vi "Write Logger.vi"(8 "error in (no error)":errorcluster, 10 "Logger":refnum<class "Logger.lvclass">, 11 "LoggingActor in":refnum<class "LoggingActor.lvclass">) -> (0 "error out":errorcluster, 3 "LoggingActor out":refnum<class "LoggingActor.lvclass">)   [LabVIEW 2022 SP3, in "LoggingActor.lvlib" / "LoggingActor.lvclass"]
uses:
  LoggingActor.lvclass
  LoggingActor.lvclass/LoggingActor.ctl
  Logger/Source/Logger/Logger.lvclass
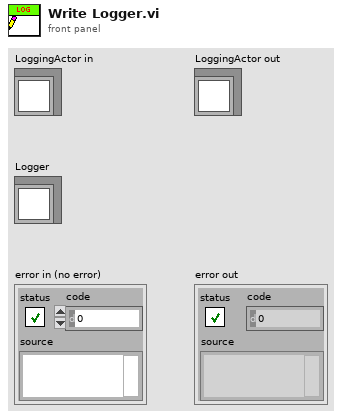
[diagram p1: front panel]
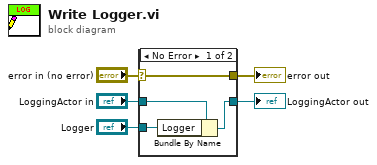
[diagram p0: block diagram]
diagram:
  n1 = case shown="No Error" "error in (no error)" {
    selector: "error in (no error)" -> [w9 w10]
    tunnel: [w9 w10] -> w4
    tunnel: [w7 w11] -> w2
    tunnel: "LoggingActor in" -> [w8 w11]
    tunnel: "Logger" -> [w6 _]
    frame No Error {
      n2 = Bundle By Name(cluster=w8, "Logger"=w6) -> (w7:refnum<class "LoggingActor.lvclass">)
    }
    frame Error {
    }
  }
  "error out" <- w4
  "LoggingActor out" <- w2
